vi "change situation.vi"(0 "pulse width":dbl, 1 "speed max":bool, 2 "speed min":bool) -> (14 "no change":bool, 15 "increas":bool, 16 "decreas":bool)   [LabVIEW 2019]
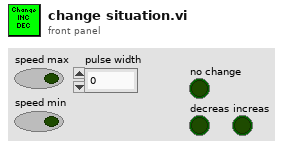
[diagram p1: front panel]
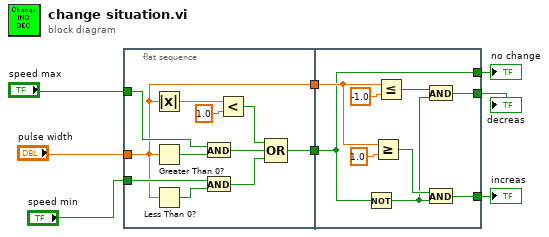
[diagram p0: block diagram]
diagram:
  n1 = flat-sequence {
    tunnel: "speed max" -> [w12]
    tunnel: "speed min" -> [w11]
    tunnel: [w13] -> w8
    tunnel: "pulse width" -> [w9]
    tunnel: [w9] -> w7
    tunnel: [w22] -> w6
    tunnel: w8 -> [w22]
    tunnel: w7 -> [w23]
    tunnel: [w21] -> w5
    tunnel: [w20] -> w4
    frame #0 {
      n2 = Absolute Value(x=w9) -> (abs(x)=w19:dbl)
      n3 = Greater Than 0?(x=w9) -> (x > 0?=w10:bool)
      n4 = Less Than 0?(x=w9) -> (x < 0?=w18:bool)
      n5 = And(x=w12, y=w10) -> (x .and. y?=w15:bool)
      n6 = And(x=w11, y=w18) -> (x .and. y?=w14:bool)
      n7 = Less?(x=w19, y=1.0) -> (x < y?=w16:bool)
      n8 = Compound Arithmetic op=OR(w16, w15, w14) -> (w13:bool)
    }
    frame #1 {
      n9 = Not(x=w22) -> (.not. x?=w27:bool)
      n10 = Greater Or Equal?(x=w23, y=1.0) -> (x >= y?=w28:bool)
      n11 = Less Or Equal?(x=w23, y=-1.0) -> (x <= y?=w26:bool)
      n12 = And(x=w26, y=w27) -> (x .and. y?=w21:bool)
      n13 = And(x=w28, y=w27) -> (x .and. y?=w20:bool)
    }
  }
  "no change" <- w6
  "decreas" <- w5
  "increas" <- w4
